vi "find_circles.vi"(5 "shrinkFactor":i32, 6 "Field of View":cluster{"fieldOfViewX":sgl, "fieldOfViewY":sgl}, 8 "error in":errorcluster, 10 "find_circles parameters":T2, 11 "Image":T3) -> (0 "error out":errorcluster, 2 "Circles":T1(array[cluster]))   [LabVIEW 2024, in "Vision.lvlib"]
uses:
  Vision.lvlib
  <vilib>/vision/Image Controls.llb/IMAQ Image.ctl
  find_circles parameters.ctl
  bin/PatternRecognition.dll
panel:
  # "Image must be an 8-bin greyscale image"
  # "For error circle"
  # "in micrometers"
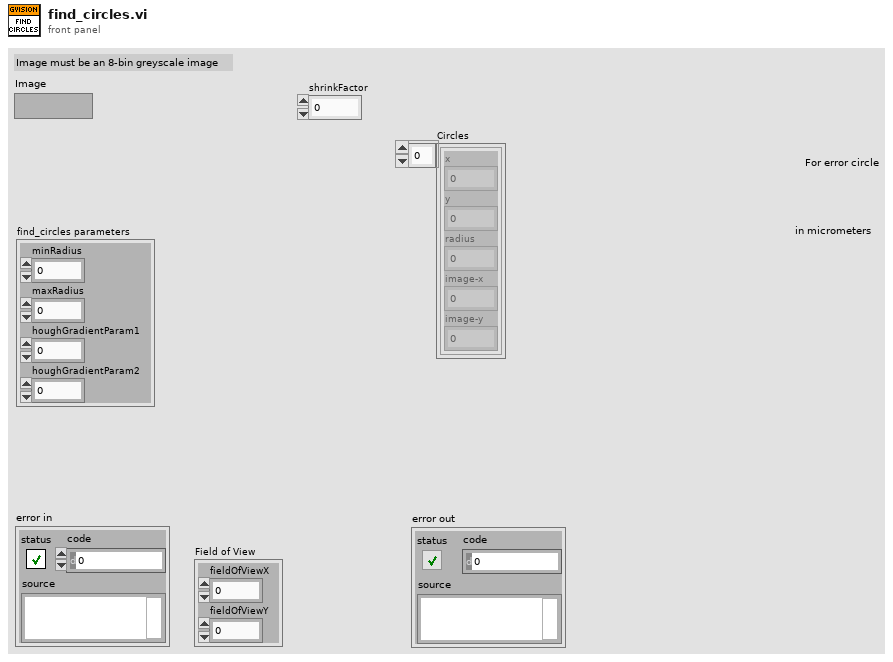
[diagram p1: front panel]
types:
  T1 = cluster{"x":dbl, "y":dbl, "radius":dbl, "image-x":dbl, "image-y":dbl}[]
  T2 = typedef "Vision.lvlib/find_circles parameters.ctl" = cluster{"minRadius":sgl, "maxRadius":sgl, "houghGradientParam1":i32, "houghGradientParam2":i32}
  T3 = typedef "IMAQ Image.ctl" = refnum<image>
  T4 = enum32{"Map Pixel Pointer", "Unmap Pixel Pointer", "Get Pixels Infos"}
  T5 = cluster{"x":dbl, "y":dbl, "radius":dbl, "image-x":dbl, "image-y":dbl}
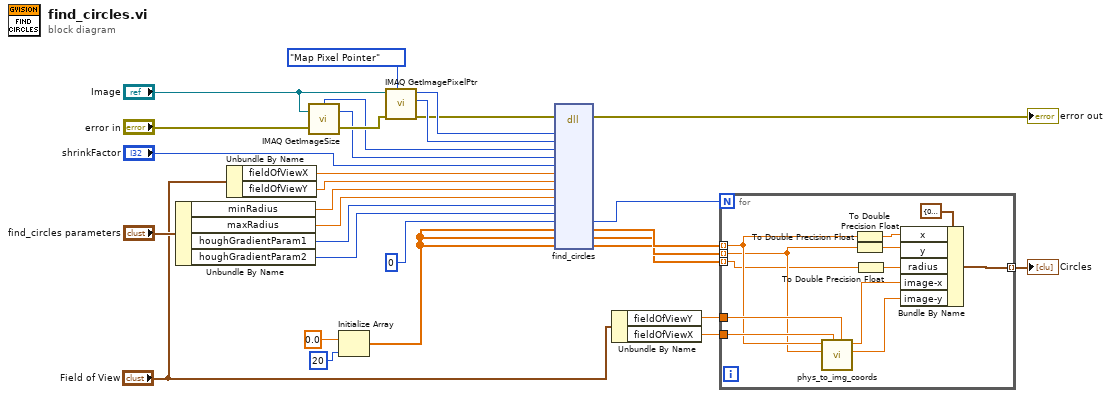
[diagram p0: block diagram]
diagram:
  n1 = Unbundle By Name("find_circles parameters") -> ("minRadius"=w21:sgl, "maxRadius"=w20:sgl, "houghGradientParam1"=w19:i32, "houghGradientParam2"=w18:i32)
  n2 = Unbundle By Name("Field of View") -> ("fieldOfViewX"=w3:sgl, "fieldOfViewY"=w2:sgl)
  n3 = call "IMAQ GetImageSize"("Image"="Image", "error in (no error)"="error in") -> ("Y Resolution"=w26:i32, "X Resolution"=w25:i32, "error out"=w27:errorcluster)  [unwired: 2 in]
  n4 = Initialize Array(sgl 0.0 ("element"), 20 ("dimension size")) -> (w15:sgl[])
  n5 = call "IMAQ GetImagePixelPtr"("Function"=T4."Map Pixel Pointer", "error in (no error)"=w27, "Image"="Image") -> ("error out"=w1:errorcluster, "LineWidth(Pixels)"=w24:i32, "Pixel Pointer out"=w23:u64)  [unwired: 3 in, 3 out]
  n6 = dll-call lib="C:/Users/cfang/Desktop/nebraska-silicon-lab/pixel-gantry-control/Gantry/Shared Components/bin/PatternRecognition.dll" fn="find_circles"(error in=w1, "img"=w23, "imgLineWidth"=w24, "imgWidth"=w25, "imgHeight"=w26, "shrinkFactor"="shrinkFactor", "fieldOfViewX"=w3, "fieldOfViewY"=w2, "minRadius"=w21, "maxRadius"=w20, "houghGradientParam1"=w19, "houghGradientParam2"=w18, "numCircles"=0, "circleXCenters"=w15, "circleYCenters"=w15, "circleRadii"=w15) -> (error out=→"error out":errorcluster, "numCircles"=w10:i32, "circleXCenters"=w9:sgl[], "circleYCenters"=w8:sgl[], "circleRadii"=w7:sgl[])  [unwired: 14 in, 1 out]
  n7 = Unbundle By Name("Field of View") -> ("fieldOfViewY"=w13:sgl, "fieldOfViewX"=w12:sgl)
  n8 = for {
    N: w10 -> [_]
    tunnel: w9 -> [w35] mode=indexing
    tunnel: w8 -> [w32] mode=indexing
    tunnel: [w42] -> w6 mode=indexing
    tunnel: w13 -> [w37]
    tunnel: w12 -> [w36]
    tunnel: w7 -> [w31] mode=indexing
    n9 = call "phys_to_img_coords.vi"("fov_y"=w37, "fov_x"=w36, "y"=w32, "x"=w35) -> ("image_y"=w33:dbl, "image_x"=w34:dbl)  [unwired: 6 in]
    n10 = To Double Precision Float(number=w35) -> (double precision float=w41:dbl)
    n11 = To Double Precision Float(number=w32) -> (double precision float=w40:dbl)
    n12 = To Double Precision Float(number=w31) -> (double precision float=w39:dbl)
    n13 = Bundle By Name(cluster=T5 {"x"=0.0, "y"=0.0, "radius"=0.0, "image-x"=0.0, "image-y"=0.0}, "x"=w41, "y"=w40, "radius"=w39, "image-x"=w34, "image-y"=w33) -> (w42:T5)
  }
  "Circles" <- w6
